vi "write TBM configuration.vi"(8 "error in":errorcluster, 10 "configuration":refnum<class "TBM configuration.lvclass">, 11 "Temperature Chamber Model editor node in":refnum<class "Temperature Chamber Model editor node.lvclass">) -> (0 "error out":errorcluster, 3 "Temperature Chamber Model editor node out":refnum<class "Temperature Chamber Model editor node.lvclass">)   [LabVIEW 2013, in "Temperature Chamber Model editor node.lvclass"]
uses:
  Temperature Chamber Model editor node.lvclass
  <vilib>/NI/Tag Bus Module Framework/root configuration/TBM configuration.lvclass
  module/configuration/Temperature Chamber Model configuration.lvclass
  Temperature Chamber Model editor node.lvclass/Temperature Chamber Model editor node.ctl
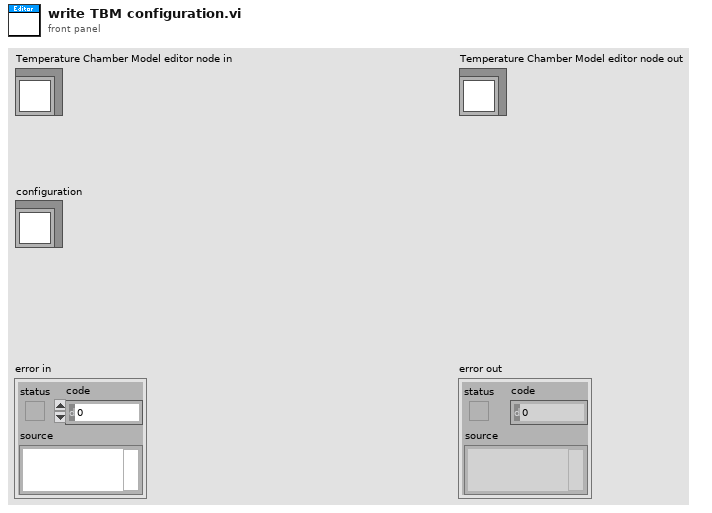
[diagram p1: front panel]
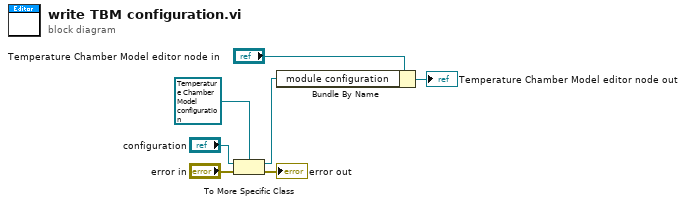
[diagram p0: block diagram]
diagram:
  n1 = To More Specific Class(target class=refnum<class "Temperature Chamber Model configuration.lvclass"> refnum ("module configuration"), reference="configuration", error in="error in") -> (specific class reference=w1:refnum<class "Temperature Chamber Model configuration.lvclass">, error out=→"error out":errorcluster)
  n2 = Bundle By Name(cluster="Temperature Chamber Model editor node in", "module configuration"=w1) -> (→"Temperature Chamber Model editor node out":refnum<class "Temperature Chamber Model editor node.lvclass">)
